vi "BoundAngleNegPiToPi.vi"(1 "angle":dbl) -> (0 "bound angle":dbl)   [LabVIEW 2015]
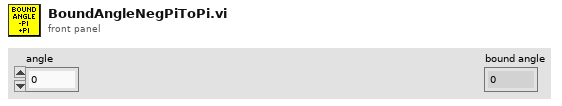
[diagram p1: front panel]
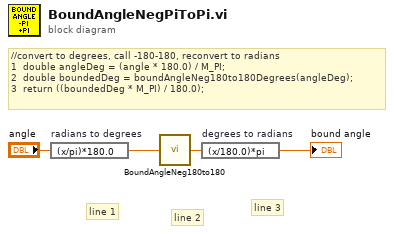
[diagram p0: block diagram]
diagram:
  # "line 3"
  # "line 2"
  # "line 1"
  # "//convert to degrees, call -180-180, reconvert to radians\n1  double angleDeg = (angle * 180.0) / M_PI;\n2  double boundedDeg = boundAngleNeg180to180Degrees(angleDeg);\n3  return ((boundedDeg * M_PI) / 180.0);"
  n1 = expression code="(x/pi)*180.0" "radians to degrees"("angle") -> (w4:dbl)
  n2 = call "BoundAngleNeg180to180.vi"("angle"=w4) -> ("bound angle"=w3:dbl)
  n3 = expression code="(x/180.0)*pi" "degrees to radians"(w3) -> (→"bound angle":dbl)
